vi "Go To Doors Closing State.vi"(8 "error in (no error)":errorcluster, 11 "Door Controller in":refnum<class "Door Controller.lvclass">) -> (0 "error out":errorcluster, 3 "Door Controller out":refnum<class "Door Controller.lvclass">)   [LabVIEW 2020, in "Door Controller.lvlib" / "Door Controller.lvclass"]
uses:
  Door Controller.lvclass
  C:/Program Files/National Instruments/LabVIEW 2020/vi.lib/ActorFramework/Actor/Actor.lvclass
  Doors Closing/Doors Closing.lvclass
  C:/Users/Thomas.McQuillan/Desktop/Elevator Door Control/State/State.lvclass
  <vilib>/ActorFramework/Actor/Actor.lvclass/Actor.ctl
  <vilib>/ActorFramework/Message Enqueuer/Message Enqueuer.lvclass/Message Enqueuer.ctl
  Door Controller Messages/Set State Msg/Set State Msg.lvclass/Set State Msg.ctl
  <vilib>/ActorFramework/Message Enqueuer/Init from Existing Queue.vi
  <vilib>/ActorFramework/Message Enqueuer/Enqueue.vi
  Door Controller Messages/Set State Msg/Set State Msg.lvclass
  C:/Program Files/National Instruments/LabVIEW 2020/vi.lib/ActorFramework/Message/Message.lvclass
  <vilib>/ActorFramework/Message Priority Queue/Priority Enqueue.vi
  <vilib>/ActorFramework/Message Enqueuer/Message Enqueuer.lvclass
  <vilib>/ActorFramework/Actor/Actor.lvclass
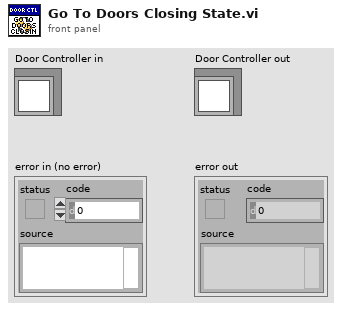
[diagram p1: front panel]
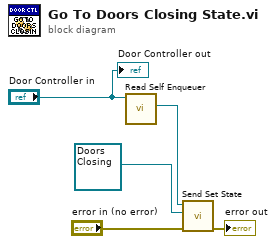
[diagram p0: block diagram]
diagram:
  n1 = call <vilib>:"Read Self Enqueuer.vi"("Actor"="Door Controller in") -> ("Self Enqueuer"=w5:refnum<class "Message Enqueuer.lvclass">)  [unwired: 10 in]
  n2 = call "Send Set State.vi"("error in (no error)"="error in (no error)", "New State In"=refnum<class "Doors Closing.lvclass"> refnum ("Door Controller.lvlib:Doors Closing.lvclass"), "Message Enqueuer"=w5) -> ("error out"=→"error out":errorcluster)  [unwired: 7 in, 1 out]
  "Door Controller out" <- "Door Controller in"
